vi "SizeMainPanel_LS1.vi"(8 "ErrorIn(No Error)":errorcluster caption="entrée d'erreur (pas d'erreur)", 11 "PaneRef":refnum<vi>) -> (0 "sortie d'erreur":errorcluster, 3 "PaneRef Out":refnum<vi>)   [LabVIEW 2019]
uses:
  <vilib>/Utility/miscctls.llb/LVPointTypeDef.ctl
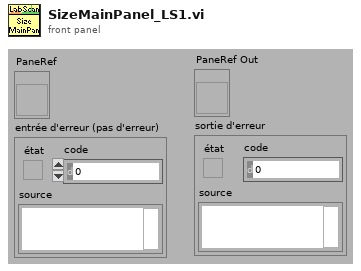
[diagram p1: front panel]
types:
  T1 = typedef "LVPointTypeDef.ctl" = cluster{"Horizontal":i16, "Vertical":i16}
  T2 = typedef "LVRectTypeDef.ctl" = cluster{"Left":i16, "Top":i16, "Right":i16, "Bottom":i16}
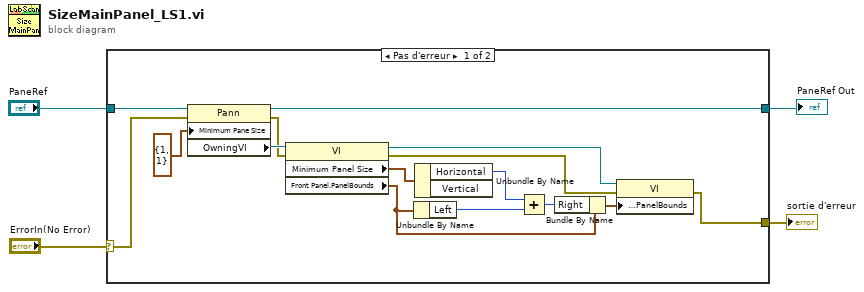
[diagram p0: block diagram]
diagram:
  n1 = case shown="Pas d'erreur" "ErrorIn(No Error)" {
    selector: "ErrorIn(No Error)" -> [w11 w21]
    tunnel: "PaneRef" -> [w19 w20]
    tunnel: [w8 w20] -> w2
    tunnel: [w7 w21] -> w1
    frame No Error {
      n2 = property class="Pann"(reference=w19, error in=w11, "Minimum Pane Size"=T1 {"Horizontal"=1, "Vertical"=1} ("Taille minimale de panneau")) -> (reference out=w8:refnum<vi>, error out=w9:errorcluster, "OwningVI"=w18:refnum<vi>)
      n3 = property class="VI"(reference=w18, error in=w9) -> (reference out=w14:refnum<vi>, error out=w10:errorcluster, "Minimum Panel Size"=w5:T1, "Front Panel.PanelBounds"=w17:T2)
      n4 = Unbundle By Name(w17) -> ("Left"=w13:i16)
      n5 = Unbundle By Name(w5) -> ("Horizontal"=w12:i16)  [unwired: 1 out]
      n6 = Add(x=w12, y=w13) -> (x+y=w16:i16)
      n7 = Bundle By Name(cluster=w17, "Right"=w16) -> (w15:T2)
      n8 = property class="VI"(reference=w14, error in=w10, "Front Panel.PanelBounds"=w15) -> (error out=w7:errorcluster)  [unwired: 1 out]
    }
    frame Error {
    }
  }
  "sortie d'erreur" <- w1
  "PaneRef Out" <- w2
